vi "GET_Running_perc._(online).vi"(8 "Reset? (F)":bool, 9 "Speed (filtered)":dbl, 10 "Histogram parameters":T2, 11 "Run time % data in":T1) -> (3 "Run time % data out":T1)   [LabVIEW 2018, in "Tracker.lvlib"]
uses:
  Tracker.lvlib
  Controls/CTL_Histogram_parameters.ctl
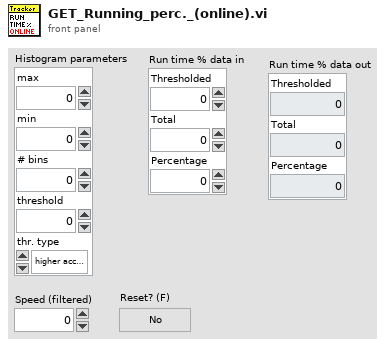
[diagram p1: front panel]
types:
  T1 = cluster{"Thresholded":u32, "Total":u32, "Percentage":dbl}
  T2 = typedef "Tracker.lvlib/CTL_Histogram_parameters.ctl" = cluster{"max":dbl, "min":dbl, "# bins":i32, "threshold":dbl, "thr. type":enum16{"higher accepted", "lower accepted"}}
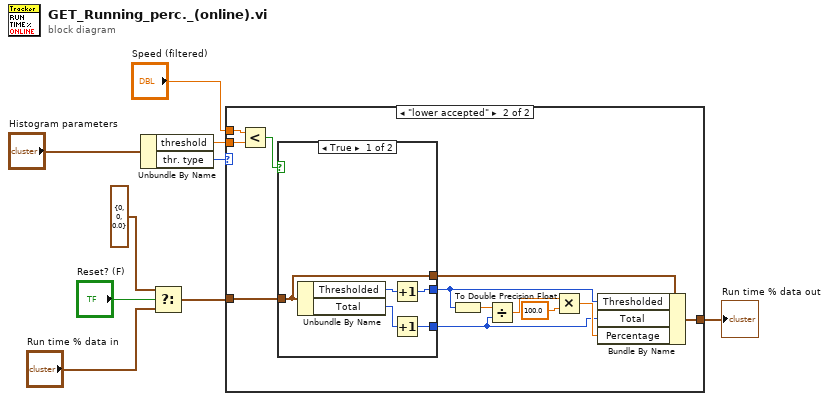
[diagram p0: block diagram]
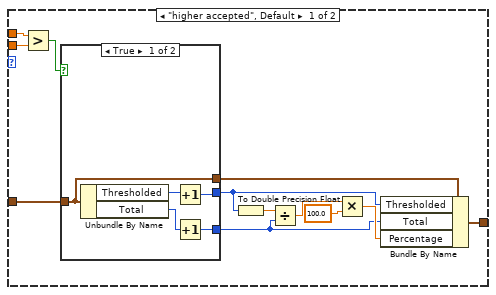
[diagram p2: hidden frame]
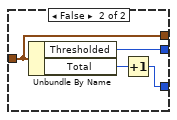
[diagram p3: hidden frame]
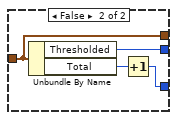
[diagram p4: hidden frame]
diagram:
  n1 = Unbundle By Name("Histogram parameters") -> ("threshold"=w6:dbl, "thr. type"=w8:enum16{"higher accepted", "lower accepted"})
  n2 = Select(t=T1 {"Thresholded"=0, "Total"=0, "Percentage"=0.0}, s="Reset? (F)", f="Run time % data in") -> (s? t:f=w5:T1)
  n3 = case shown="\"lower accepted\"" w8 {
    tunnel: "Speed (filtered)" -> [w21 w42]
    tunnel: w6 -> [w20 w41]
    tunnel: w5 -> [w15 w36]
    tunnel: [w10 w31] -> w1
    frame "higher accepted", Default {
      n4 = Greater?(x=w21, y=w20) -> (0:w19:bool)
      n5 = case shown="True" w19 {
        tunnel: w15 -> [w22 w27]
        tunnel: [w24 w29] -> w12
        tunnel: [w23 w28] -> w11
        tunnel: [w22 w27] -> w14
        frame True {
          n6 = Unbundle By Name(w22) -> ("Thresholded"=w26:u32, "Total"=w25:u32)
          n7 = Increment(x=w26) -> (x+1=w23:u32)
          n8 = Increment(x=w25) -> (x+1=w24:u32)
        }
        frame False {
          n9 = Unbundle By Name(w27) -> ("Thresholded"=w28:u32, "Total"=w30:u32)
          n10 = Increment(x=w30) -> (x+1=w29:u32)
        }
      }
      n11 = To Double Precision Float(number=w11) -> (double precision float=w18:dbl)
      n12 = Divide(x=w18, y=w12) -> (x/y=w17:dbl)
      n13 = Multiply(x=w17, y=100.0) -> (x*y=w13:dbl)
      n14 = Bundle By Name(cluster=w14, "Thresholded"=w11, "Total"=w12, "Percentage"=w13) -> (w10:T1)
    }
    frame "lower accepted" {
      n15 = Less?(x=w42, y=w41) -> (x < y?=w40:bool)
      n16 = case shown="True" w40 {
        tunnel: w36 -> [w43 w48]
        tunnel: [w45 w50] -> w33
        tunnel: [w44 w49] -> w32
        tunnel: [w43 w48] -> w35
        frame True {
          n17 = Unbundle By Name(w43) -> ("Thresholded"=w47:u32, "Total"=w46:u32)
          n18 = Increment(x=w47) -> (x+1=w44:u32)
          n19 = Increment(x=w46) -> (x+1=w45:u32)
        }
        frame False {
          n20 = Unbundle By Name(w48) -> ("Thresholded"=w49:u32, "Total"=w51:u32)
          n21 = Increment(x=w51) -> (x+1=w50:u32)
        }
      }
      n22 = To Double Precision Float(number=w32) -> (double precision float=w39:dbl)
      n23 = Divide(x=w39, y=w33) -> (x/y=w38:dbl)
      n24 = Multiply(x=w38, y=100.0) -> (x*y=w34:dbl)
      n25 = Bundle By Name(cluster=w35, "Thresholded"=w32, "Total"=w33, "Percentage"=w34) -> (w31:T1)
    }
  }
  "Run time % data out" <- w1
